vi "Transfer Line Status.vi"(8 "error in (no error)":errorcluster, 11 "Vacuum in":refnum<class "Vacuum.lvclass">) -> (0 "error out":errorcluster, 3 "Vacuum out":refnum<class "Vacuum.lvclass">)   [LabVIEW 2015, in "AMS UI.lvlib" / "Vacuum.lvclass"]
uses:
  Vacuum.lvclass
  Controls/Ti Colors.ctl
  AMS Gas Messages/Set Transfer Line Color Msg/Set Transfer Line Color Msg.lvclass/Set Transfer Line Color Msg.ctl
  <vilib>/ActorFramework/Message Enqueuer/Message Enqueuer.lvclass/Message Enqueuer.ctl
  <vilib>/ActorFramework/Message Enqueuer/Enqueue.vi
  <vilib>/ActorFramework/Message Priority Queue/Priority Enqueue.vi
  AMS Gas Messages/Set Transfer Line Color Msg/Set Transfer Line Color Msg.lvclass
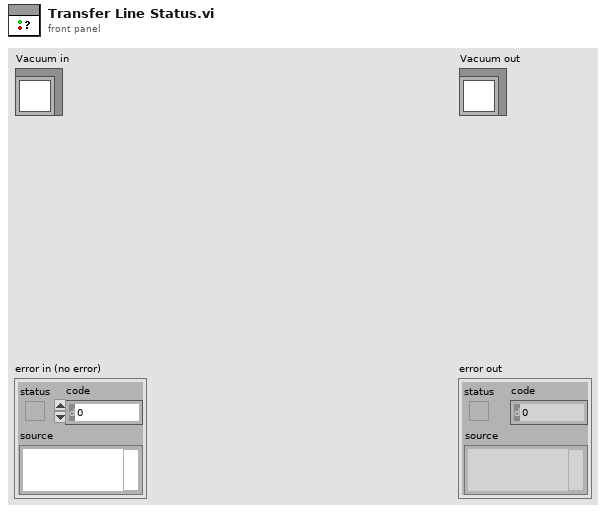
[diagram p1: front panel]
types:
  T1 = typedef "Ti Colors.ctl" = u32[]
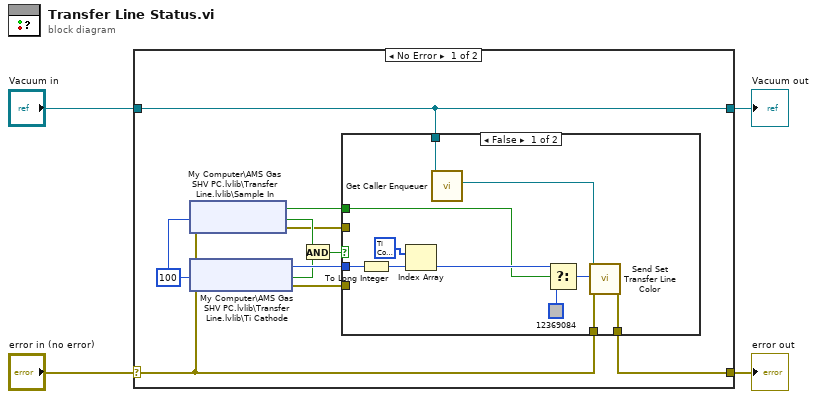
[diagram p0: block diagram]
diagram:
  n1 = case shown="No Error" "error in (no error)" {
    selector: "error in (no error)" -> [w11 w29]
    tunnel: [w14 w29] -> w3
    tunnel: [w15 w28] -> w1
    tunnel: "Vacuum in" -> [w15 w28]
    frame No Error {
      w10 = 100 ("ms timeout (0)")
      n2 = shared-variable "My Computer\\AMS Gas SHV PC.lvlib\\Transfer Line.lvlib\\Sample In"(error in=w11, w10) -> (w5:bool, error out=w6:errorcluster, w7:bool)
      n3 = shared-variable "My Computer\\AMS Gas SHV PC.lvlib\\Transfer Line.lvlib\\Ti Cathode"(error in=w11, w10) -> (w12:i8, error out=w13:errorcluster, w9:bool)
      n4 = And(x=w7, y=w9) -> (x .and. y?=w8:bool)
      n5 = case shown="False" w8 {
        tunnel: w15 -> [w25 _]
        tunnel: w11 -> [w24 w27]
        tunnel: [w23 w27] -> w14
        tunnel: w13 -> [_ _]
        tunnel: w12 -> [w20 _]
        tunnel: w6 -> [_ _]
        tunnel: w5 -> [w16 _]
        frame False {
          n6 = To Long Integer(number=w20) -> (32bit integer=w19:i32)
          n7 = Index Array(array=T1 [418898, 837796, 1256694, 1675592, 2094490, 2513388, 2932286, 3351184, 3770082, 4188980, 4607878, 5026776, 5445674, 5864572, 6283470, 6702368, 7121266, 7540164, 7959062, 8377960, 8796858, 9215756, 9634654, 10053552, 10472450, 10891348, 11310246, 11729144, 12148042, 12566940, 12985838, 13404736, 13823634, 14242532, 14661430, 15080328, 15499226, 15918124, 16337022, 16755920] ("output array 2"), index=w19) -> (element=w17:u32)
          n8 = call-dynamic "Get Caller Enqueuer.vi"("eActor in"=w25) -> ("Actor Framework:Message Enqueuer"=w26:refnum<class "Message Enqueuer.lvclass">)  [unwired: 9 in, 1 out]
          n9 = Select(t=w17, s=w16, f=u32 12369084 ("Round Color Box")) -> (s? t:f=w22:u32)
          n10 = call "Send Set Transfer Line Color.vi"("error in (no error)"=w24, "Round Color Box"=w22, "Message Enqueuer"=w26) -> ("error out"=w23:errorcluster)  [unwired: 7 in, 1 out]
        }
        frame True {
        }
      }
    }
    frame Error {
    }
  }
  "error out" <- w3
  "Vacuum out" <- w1
